vi "fact.vi"(1 "N":i32) -> (0 "N !":u64)   [LabVIEW 2017]
doc: "Расчитывает N!\n\n0!=1 по определению\nДля N=1,2,3,...\nN!=1*2*...*N\nN!=(N-1)!*N"
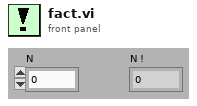
[diagram p1: front panel]
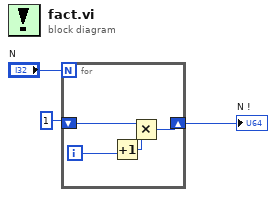
[diagram p0: block diagram]
diagram:
  n1 = for {
    N: "N" -> [_]
    shift-right: [w5] -> w2
    shift-left: u64 1 -> [w7]
    i -> [w4]
    n2 = Increment(x=w4) -> (x+1=w6:i32)
    n3 = Multiply(x=w7, y=w6) -> (x*y=w5:u64)
  }
  "N !" <- w2
